vi "Format Entry.vi"(8 "error in (no error)":errorcluster, 10 "Log Data":T1={"Time"=timestamp(0 s since 1904-01-01), "Level"=enum."INFO", "Logger"="", "Message"="", "Arguments"=[]} {"Time" format="%<%x %.3X>T"}, 11 "Layout in":refnum<class "Layout.lvclass">) -> (0 "error out":errorcluster, 2 "Log Entry":string, 3 "Layout out":refnum<class "Layout.lvclass">)   [LabVIEW 2019, in "TSC Event Logger.lvlib" / "Layout.lvclass"]
doc: "Format the Log Entry method.\n\n<b>Code Developed By:</b>\nTechnology Service Corporation\nBloomington, IN 47403\nwww.tsc.com/atcs\n\nDeveloper:\nDaniel Coons"
uses:
  Layout.lvclass
  Log Data.ctl
  Log/Event Level.ctl
  TSC Event Logger.lvlib
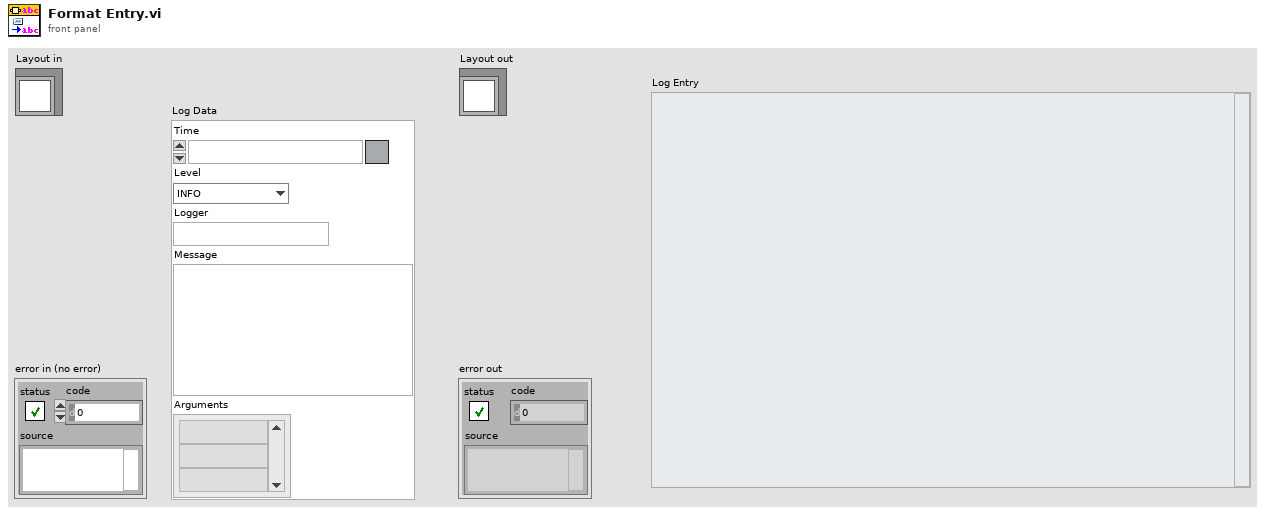
[diagram p1: front panel]
types:
  T1 = typedef "TSC Event Logger.lvlib/Log Data.ctl" = cluster{"Time":timestamp, "Level":T2, "Logger":string, "Message":string, "Arguments":string[]}
  T2 = typedef "TSC Event Logger.lvlib/Event Level.ctl" = enum16{"OFF", "TRACE", "DEBUG", "INFO", "WARN", "ERROR", "FATAL"}
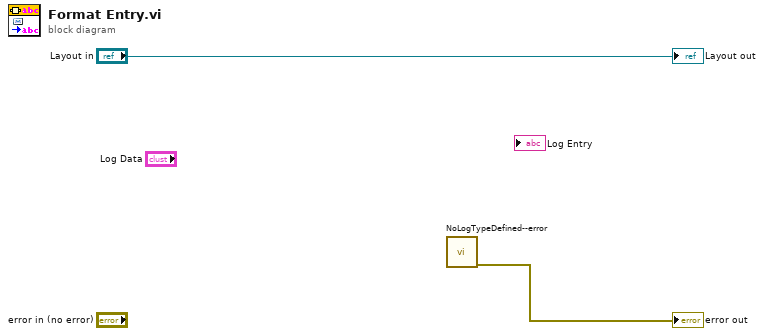
[diagram p0: block diagram]
diagram:
  n1 = call "NoLogTypeDefined--error.vi"() -> ("Error Out"=→"error out":errorcluster)  [unwired: 11 in]
  "Layout out" <- "Layout in"
